vi "CSM - Synchronized Call.vi"   [LabVIEW 2020, in "Communicable State Machine.lvlib"]
doc: "VI snippet for dropping sync call template code from LabVIEW Quick Drop.\n\n<b>Inputs:</b>\n - N/A\n -\n<b>Outputs:</b>\n - N/A"
uses:
  Communicable State Machine.lvlib
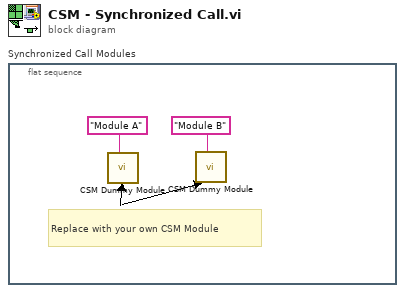
[diagram p0: block diagram]
diagram:
  n1 = flat-sequence "Synchronized Call Modules" {
    frame #0 {
      # "Replace with your own CSM Module"
      n2 = call "CSM Dummy Module.vi"("Name(\"\" to use uuid)"="Module A" ("Name(\"\" to use uuid)")) -> ()  [unwired: 11 in]
      n3 = call "CSM Dummy Module.vi"("Name(\"\" to use uuid)"="Module B" ("Name(\"\" to use uuid)")) -> ()  [unwired: 11 in]
    }
  }
